vi "create incident - command.vi"(8 "data":variant, 9 "command":string, 11 "RT Queues":T1) -> ()   [LabVIEW 2018]
uses:
  Type Defs/Queues cluster.ctl
  Chris VIs/Message Scheduler/message scheduler.lvclass
  Type Defs/generic incident.ctl
  Queue VIs/En-queue RT comms element.vi
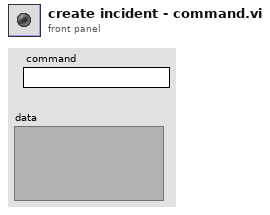
[diagram p1: front panel]
types:
  T1 = typedef "Queues cluster.ctl" = cluster{"RT Message":refnum<queue>, "RT Comms":refnum<queue>, "RT Data":refnum<queue>, "RT FIFO":refnum<queue>, "message scheduler":refnum<class "message scheduler.lvclass">}
  T2 = typedef "generic incident.ctl" = cluster{"timestamp":timestamp, "type":string, "Variant":variant}
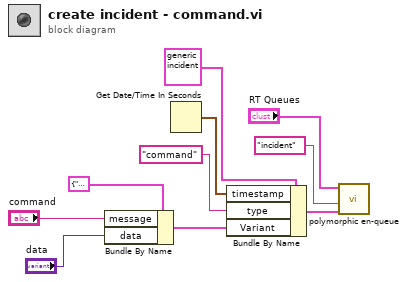
[diagram p0: block diagram]
diagram:
  n1 = Bundle By Name(cluster=cluster{"message":string, "data":variant} {"message"="", "data"=variant}, "message"="command", "data"="data") -> (w8:cluster{"message":string, "data":variant})
  n2 = Get Date/Time In Seconds() -> (seconds since 1Jan1904=w5:timestamp)
  n3 = Bundle By Name(cluster=T2 {"timestamp"=timestamp(0 s since 1904-01-01), "type"="", "Variant"=variant} ("incident cluster"), "timestamp"=w5, "type"="command", "Variant"=w8) -> (w4:T2)
  n4 = call-poly "polymorphic en-queue.vi"("Data"=w4, "Message"="incident", "RT Queues"="RT Queues") -> ()  [unwired: 8 in, 1 out]
